vi "SLSC Convert Tree Item Tag to Channel Name.vi"(10 "Type of Item":string="/Properties", 11 "Item String":string) -> (1 "Item Name":string, 2 "Type of Item":string, 3 "Device/Physical Channel":string)   [LabVIEW 2017, in "SLSC Tree Control.lvlib"]
uses:
  SLSC Tree Control.lvlib
  <vilib>/regexp/Match Regular Expression.xnode
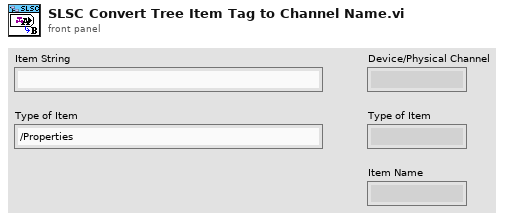
[diagram p1: front panel]
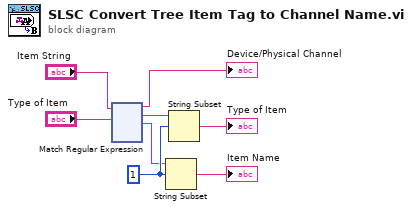
[diagram p0: block diagram]
diagram:
  w6 = 1 ("offset (0)")
  n1 = xnode "Match Regular Expression"("input string"="Item String", "regular expression"="Type of Item") -> ("before match"=→"Device/Physical Channel":string, "whole match"=w7:string, "after match"=w5:string)  [unwired: 4 in, 2 out]
  n2 = String Subset(string=w5, offset (0)=w6) -> (substring=→"Item Name":string)  [unwired: 1 in]
  n3 = String Subset(string=w7, offset (0)=w6) -> (substring=→"Type of Item":string)  [unwired: 1 in]
